vi "LV SciSDK TOF SPECTRUM START.vi"(0 "TOF Spectrum Name":string, 5 "Bin Width":u32, 7 "Start Delay":u32, 9 "Board Handle In":T1, 11 "error in (no error)":errorcluster) -> (8 "TOF Spectrum Handle Out":T2, 10 "Board Handle Out":T1, 15 "error out":errorcluster)   [LabVIEW 2021, in "SciSDK_Labview.lvlib"]
doc: "You need this VI to execute 'start' spectrum component command"
uses:
  SciSDK_Labview.lvlib
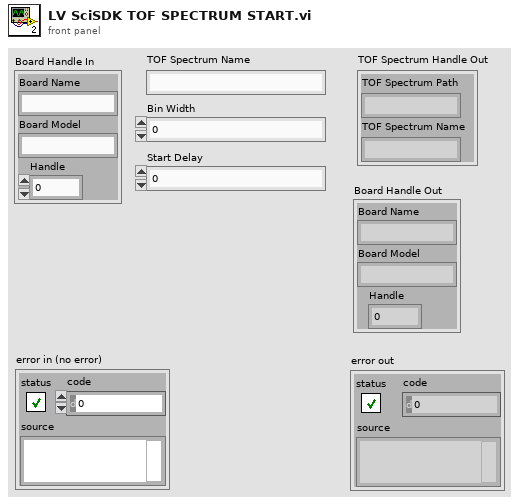
[diagram p1: front panel]
types:
  T1 = cluster{"Board Name":string, "Board Model":string, "Handle":u64}
  T2 = cluster{"TOF Spectrum Path":string, "TOF Spectrum Name":string}
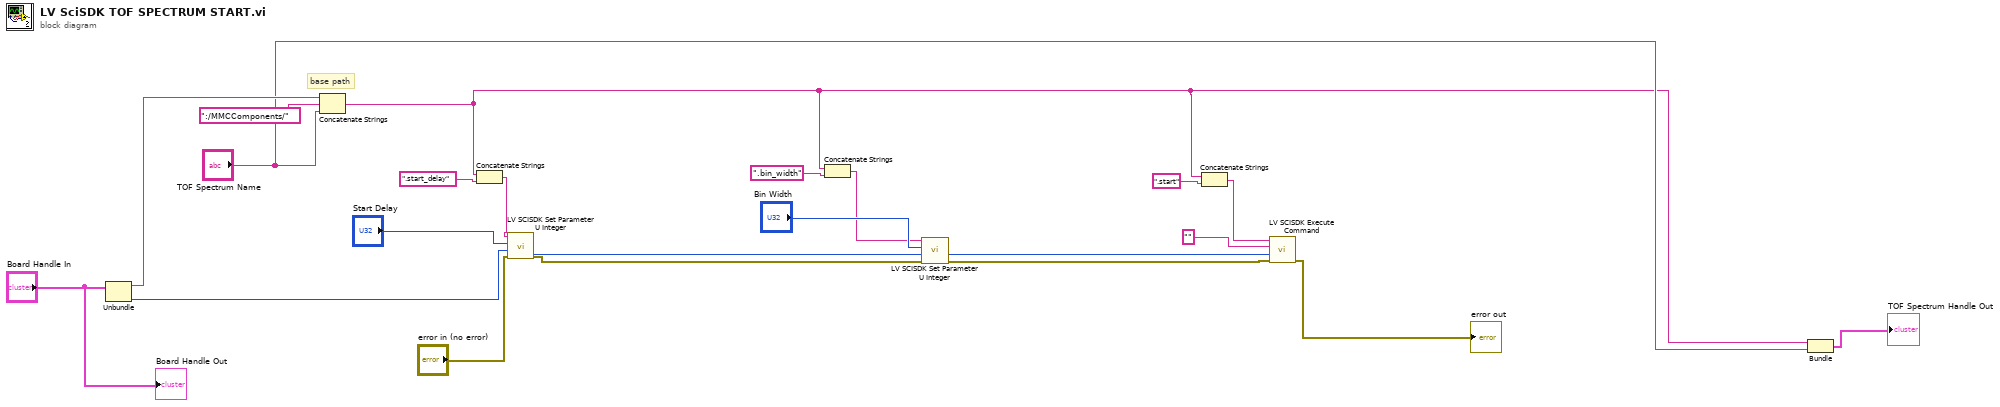
[diagram p0: block diagram]
diagram:
  # "base path"
  n1 = Unbundle("Board Handle In") -> ("Board Name"=w21:string, "Handle"=w11:u64)  [unwired: 1 out]
  n2 = Concatenate Strings(w21, ":/MMCComponents/" ("string"), "TOF Spectrum Name") -> (w2:string)
  n3 = Concatenate Strings(w2, ".start_delay" ("string")) -> (w14:string)
  n4 = call "LV SCISDK Set Parameter U Integer.vi"("error in (no error)"="error in (no error)", "handle"=w11, "value"="Start Delay", "Path"=w14) -> ("error out"=w9:errorcluster, "handle out"=w12:u64)  [unwired: 5 in, 1 out]
  n5 = Concatenate Strings(w2, ".bin_width" ("string")) -> (w13:string)
  n6 = call "LV SCISDK Set Parameter U Integer.vi"("error in (no error)"=w9, "handle"=w12, "value"="Bin Width", "Path"=w13) -> ("error out"=w8:errorcluster, "handle out"=w7:u64)  [unwired: 5 in, 1 out]
  n7 = Concatenate Strings(w2, ".start" ("string")) -> (w4:string)
  n8 = call "LV SCISDK Execute Command.vi"("error in (no error)"=w8, "handle"=w7, "value"="" ("concatenated string"), "Path"=w4) -> ("error out"=→"error out":errorcluster)  [unwired: 5 in, 2 out]
  n9 = Bundle(w2, "TOF Spectrum Name"="TOF Spectrum Name") -> (→"TOF Spectrum Handle Out":cluster{string, "TOF Spectrum Name":string})  [unwired: 1 in]
  "Board Handle Out" <- "Board Handle In"
